vi "Update DAQ Parameters.vi"(8 "error in (no error)":errorcluster, 11 "DAQ Class in":refnum<class "DAQ Class.lvclass">=refnum) -> (0 "error out":errorcluster, 2 "DAQ Parameters Out":T1={"Points Per A-Scan"=1280, "A-Scans Per B-Scan"=512, "Number of B-Scans"=1, "B-Scans Per Transfer"=1024, "Trigger Voltage"=140.0, "Trigger Source"=enum."External", "Trigger Slope"=enum."Rising", "Channel"=enum."Channel 1", "Clock"=enum."External Clock", "Bits per Sample"=16.0, "Range"=4.0, "Start Trim"=140, "Stop Trim"=140}, 3 "DAQ Class out":refnum<class "DAQ Class.lvclass">)   [LabVIEW 2015, in "DAQ Class.lvclass"]
uses:
  DAQ Class.lvclass
  ATS9350/ATS9350.lvclass
  DAQ Parameters.ctl
  Trigger Source.ctl
  Trigger Slope.ctl
  Type Defs/OCT DAQ Channel Data Type.ctl
  Clock Control.ctl
panel:
  in  "DAQ Parameters":T1={"Points Per A-Scan"=1280, "A-Scans Per B-Scan"=250, "Number of B-Scans"=1, "B-Scans Per Transfer"=2, "Trigger Voltage"=140.0, "Trigger Source"=enum."External", "Trigger Slope"=enum."Rising", "Channel"=enum."Channel 1", "Clock"=enum."External Clock", "Bits per Sample"=16.0, "Range"=4.0, "Start Trim"=0, "Stop Trim"=0}
  in  "OK Button":bool
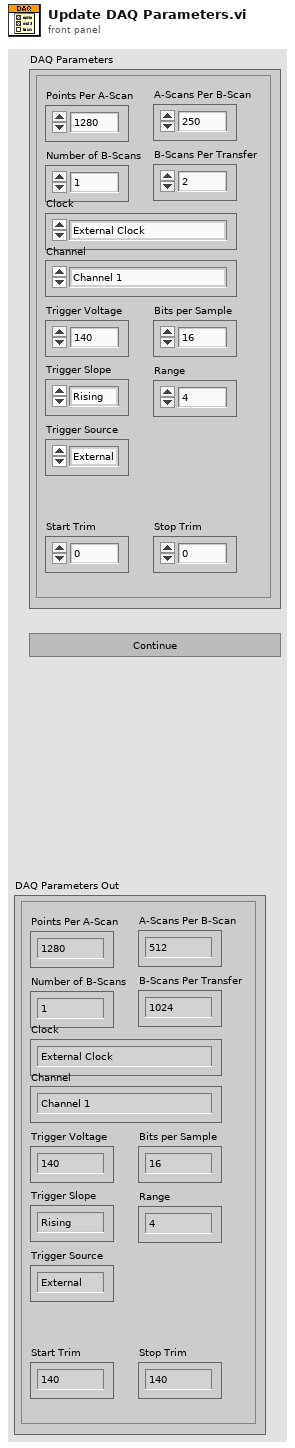
[diagram p1: front panel]
types:
  T1 = typedef "DAQ Class.lvclass/DAQ Parameters.ctl" = cluster{"Points Per A-Scan":u32, "A-Scans Per B-Scan":u32, "Number of B-Scans":u32, "B-Scans Per Transfer":u32, "Trigger Voltage":sgl, "Trigger Source":T2, "Trigger Slope":T3, "Channel":T4, "Clock":T5, "Bits per Sample":dbl, "Range":dbl, "Start Trim":u32, "Stop Trim":u32}
  T2 = typedef "DAQ Class.lvclass/Trigger Source.ctl" = enum16{"External", "Channel A", "Channel B"}
  T3 = typedef "DAQ Class.lvclass/Trigger Slope.ctl" = enum16{"Rising", "Falling"}
  T4 = typedef "OCT DAQ Channel Data Type.ctl" = enum16{"Channel 1", "Channel 2", "Channel 1 and 2"}
  T5 = typedef "DAQ Class.lvclass/Clock Control.ctl" = enum16{"Internal Clock", "External Clock"}
  T6 = enum8{"Enabled", "Disabled", "Disabled and Grayed Out"}
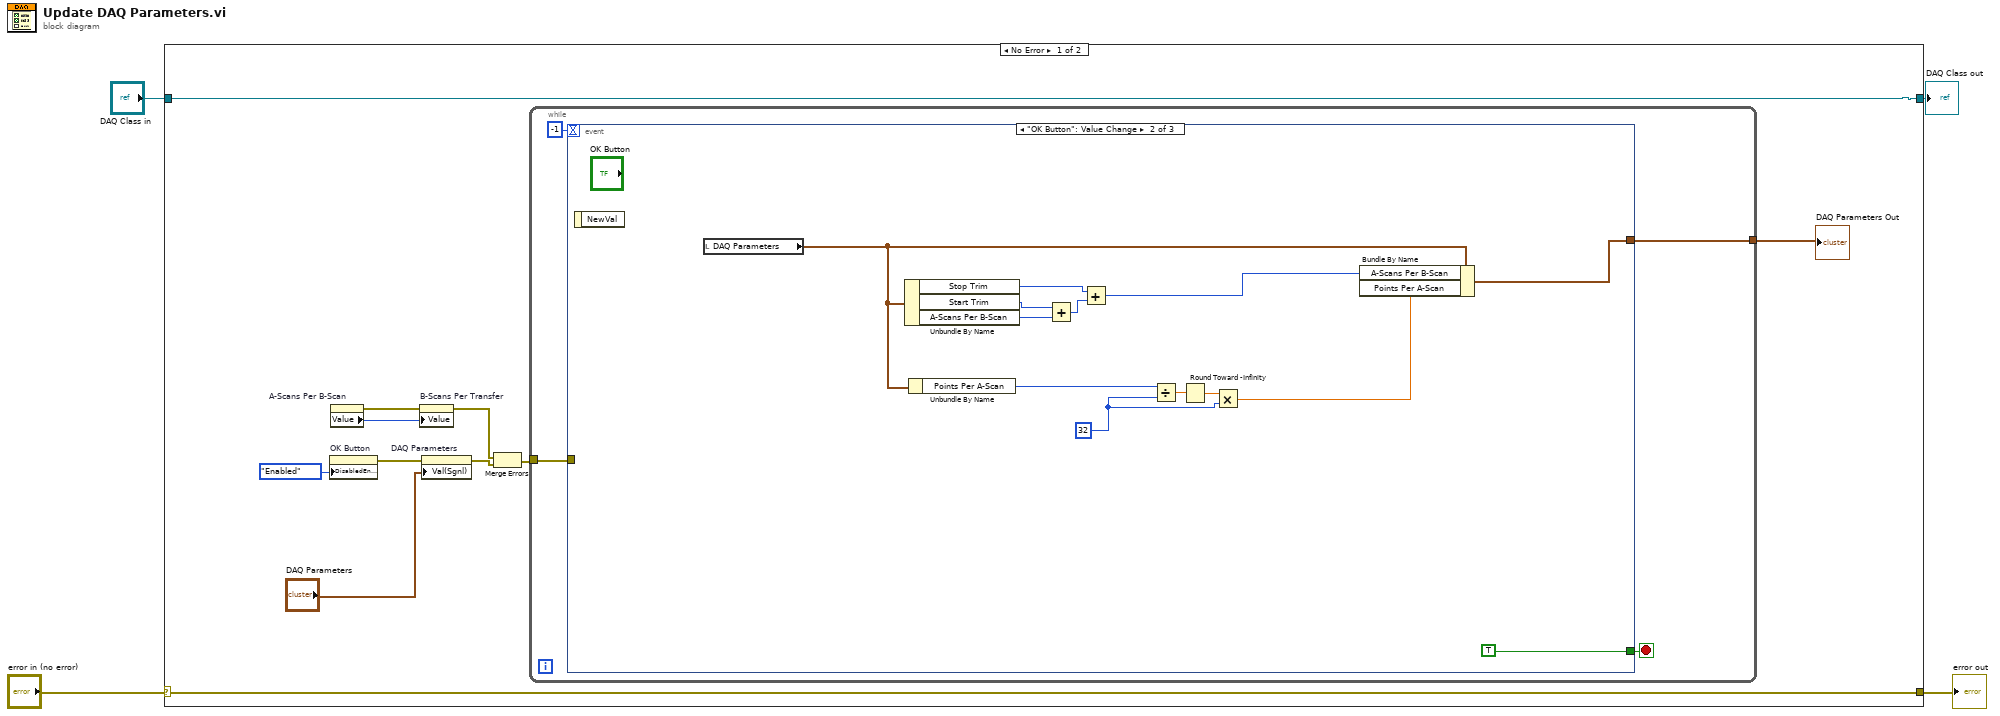
[diagram p0: block diagram]
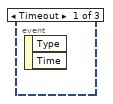
[diagram p2: hidden frame]
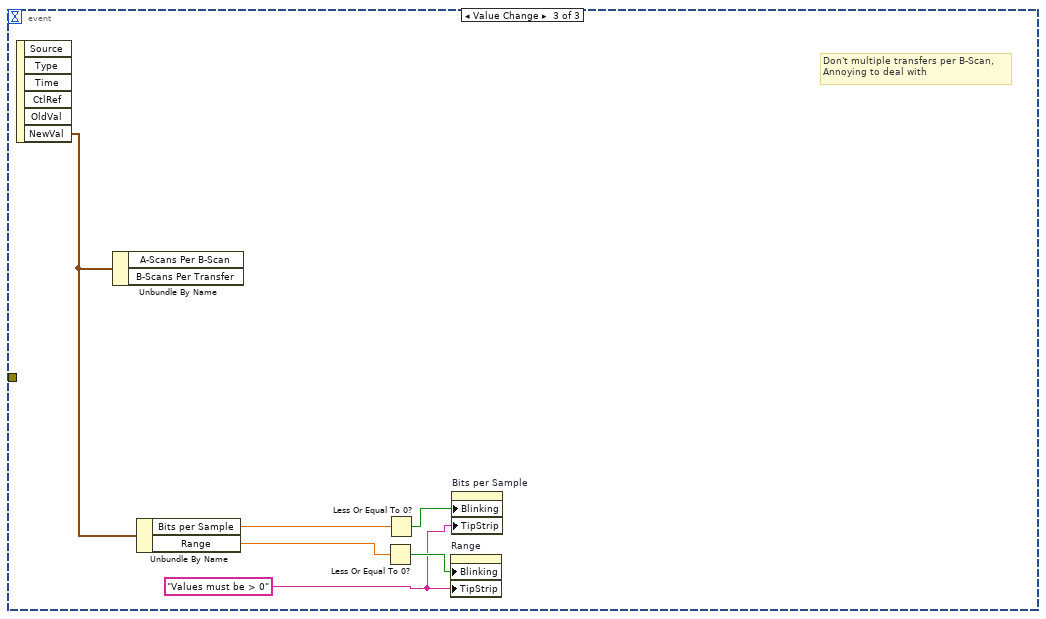
[diagram p3: hidden frame]
diagram:
  n1 = case shown="No Error" "error in (no error)" {
    selector: "error in (no error)" -> [w15 w40]
    tunnel: [w15 w40] -> w3
    tunnel: [w14 w39] -> w1
    tunnel: "DAQ Class in" -> [w14 w39]
    frame No Error {
      n2 = property on="OK Button" class="Bool"("DisabledEnum"=T6."Enabled" ("Disabled")) -> (error out=w11:errorcluster)  [unwired: 2 in, 1 out]
      n3 = property on="A-Scans Per B-Scan" class="DigNum (strict)"() -> (error out=w10:errorcluster, "Value"=w9:u32)  [unwired: 2 in, 1 out]
      n4 = property on="B-Scans Per Transfer" class="DigNum (strict)"(error in=w10, "Value"=w9) -> (error out=w7:errorcluster)  [unwired: 1 in, 1 out]
      n5 = property on="DAQ Parameters" class="Clust (strict)"(error in=w11, "Val(Sgnl)"="DAQ Parameters") -> (error out=w8:errorcluster)  [unwired: 1 in, 1 out]
      n6 = Merge Errors(w7, w8) -> (w6:errorcluster)
      n7 = while {
        tunnel: [w17] -> w13
        tunnel: w6 -> [w16]
        stop <- w18 stop-if-true
        n8 = event shown="[1] \"OK Button\": Value Change" {
          selector: _ -> [_ _ _]
          dyn-events: _ -> [_ _ _]
          timeout: -1 -> [_ _ _]
          tunnel: [_ TRUE _] -> w18
          tunnel: [_ w27 _] -> w17
          tunnel: w16 -> [_ _ _]
          event Timeout {
            n9 = event-data() -> ()  [unwired: 1 in, 2 out]
          }
          event "OK Button": Value Change {
            w23 = u32 32 ("y")
            n10 = event-data() -> ()  [unwired: 1 in, 1 out]
            n11 = local read "DAQ Parameters"() -> (w22:T1)
            n12 = Unbundle By Name(w22) -> ("Stop Trim"=w28:u32, "Start Trim"=w30:u32, "A-Scans Per B-Scan"=w31:u32)
            n13 = Unbundle By Name(w22) -> ("Points Per A-Scan"=w21:u32)
            n14 = Add(x=w30, y=w31) -> (x+y=w29:u32)
            n15 = Add(x=w28, y=w29) -> (x+y=w26:u32)
            n16 = Divide(x=w21, y=w23) -> (x/y=w25:dbl)
            n17 = Round Toward -Infinity(1:w25) -> (0:w24:dbl)
            n18 = Multiply(x=w24, y=w23) -> (x*y=w20:dbl)
            n19 = Bundle By Name(cluster=w22, "A-Scans Per B-Scan"=w26, "Points Per A-Scan"=w20) -> (w27:T1)
          }
          event Value Change {
            w33 = "Values must be > 0" ("Tip Strip")
            # "Don't multiple transfers per B-Scan,\nAnnoying to deal with"
            n20 = event-data() -> ("NewVal"=w38:T1)  [unwired: 1 in, 5 out]
            n21 = Unbundle By Name(w38) -> ()  [unwired: 2 out]
            n22 = Unbundle By Name(w38) -> ("Bits per Sample"=w37:dbl, "Range"=w36:dbl)
            n23 = Less Or Equal To 0?(x=w36) -> (x <= 0?=w34:bool)
            n24 = Less Or Equal To 0?(x=w37) -> (x <= 0?=w35:bool)
            n25 = property on="Range" class="DigNum (strict)"("Blinking"=w34, "TipStrip"=w33) -> ()  [unwired: 2 in, 2 out]
            n26 = property on="Bits per Sample" class="DigNum (strict)"("Blinking"=w35, "TipStrip"=w33) -> ()  [unwired: 2 in, 2 out]
          }
        }
      }
      "DAQ Parameters Out" <- w13
    }
    frame Error {
    }
  }
  "error out" <- w3
  "DAQ Class out" <- w1
